vi "FSK_GenBit.vi"(8 "error in (no error)":errorcluster caption="错误输入（无错误）", 11 "PathIn":path) -> (0 "error out":errorcluster caption="错误输出", 2 "SendBit":dbl[](array[numeric]) format="%#_13g", 3 "PathOut":path)   [LabVIEW 2015]
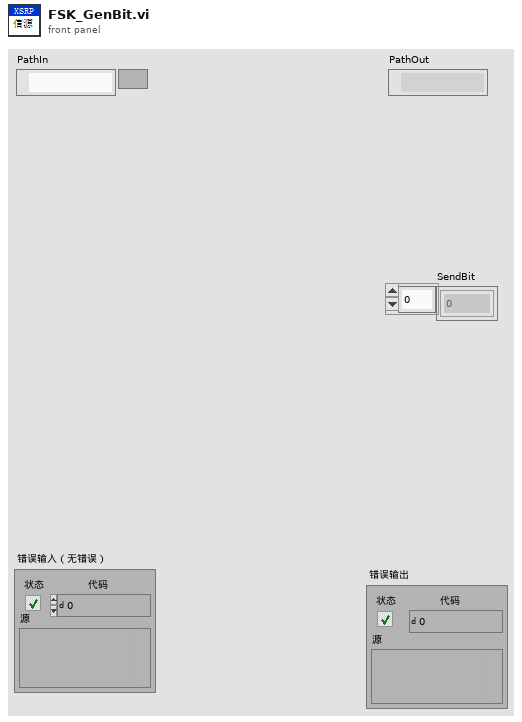
[diagram p1: front panel]
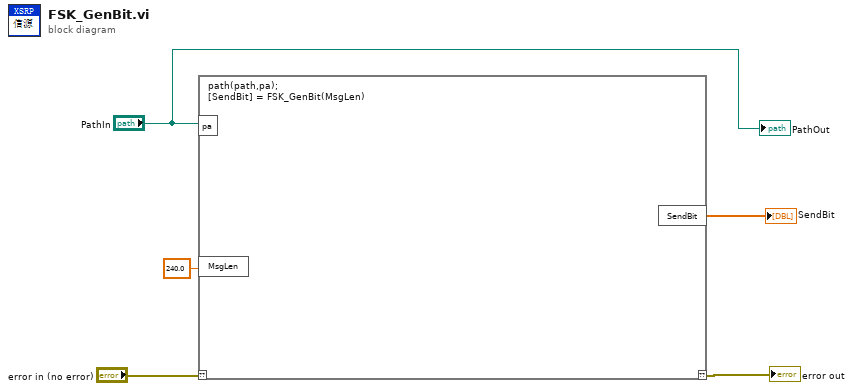
[diagram p0: block diagram]
diagram:
  n1 = script code="path(path,pa);\n[SendBit] = FSK_GenBit(MsgLen)"("??"="error in (no error)", "pa"="PathIn", "MsgLen"=240.0) -> ("??"=→"error out":errorcluster, "SendBit"=→"SendBit":dbl[])
  "PathOut" <- "PathIn"
